vi "food.vi"(0 "reference":refnum<vi>) -> ()   [LabVIEW 2009]
uses:
  Control 3.ctl
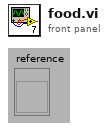
[diagram p1: front panel]
types:
  T1 = typedef "Control 3.ctl" = bool
  T2 = typedef "Control 3" = bool
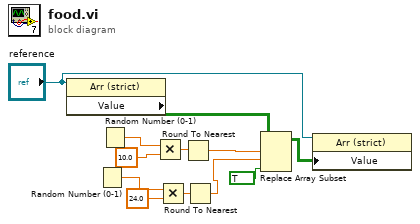
[diagram p0: block diagram]
diagram:
  n1 = property class="Arr (strict)"(reference="reference") -> ("Value"=w3:T2[][])  [unwired: 1 in, 2 out]
  n2 = Random Number (0-1)() -> (number: 0 to 1=w7:dbl)
  n3 = Random Number (0-1)() -> (number: 0 to 1=w6:dbl)
  n4 = Multiply(x=w6, y=10.0) -> (x*y=w9:dbl)
  n5 = Multiply(x=w7, y=24.0) -> (x*y=w5:dbl)
  n6 = Round To Nearest(number=w9) -> (nearest integer value=w10:dbl)
  n7 = Round To Nearest(number=w5) -> (nearest integer value=w4:dbl)
  n8 = Replace Array Subset(array=w3, new element=T1 TRUE ("new element/subarray"), index (row)=w10, index (col)=w4) -> (w2:T2[][])
  n9 = property class="Arr (strict)"(reference="reference", "Value"=w2) -> ()  [unwired: 1 in, 2 out]
